vi "set led.vi"(8 "error in (no error)":errorcluster, 10 "state":i32, 11 "led":u32(ring) items=["GREEN", "RED"]) -> (0 "error out":errorcluster, 3 "function return":i32)   [LabVIEW 2014, in "libroboticscape.lvlib"]
doc: "int set_led(led_t led, int state);"
uses:
  libroboticscape.lvlib
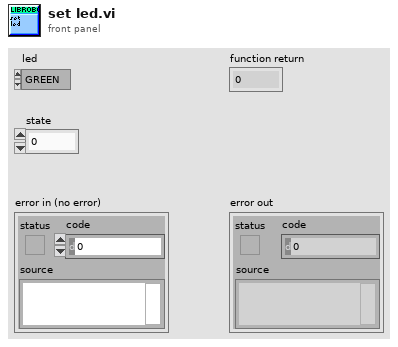
[diagram p1: front panel]
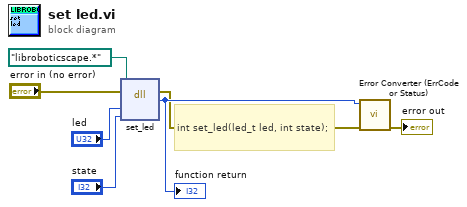
[diagram p0: block diagram]
diagram:
  # "int set_led(led_t led, int state);"
  n1 = dll-call lib="C:/Users/ktalke/Documents/Robotics-Cape-Master-Jessie/Libroboticscape-Master-Jessie/libroboticscape.so" fn="set_led"(path in=path "libroboticscape.*", error in="error in (no error)", "led"="led", "state"="state") -> (error out=w3:errorcluster, "return type"=w7:i32)  [unwired: 3 in, 1 out]
  "function return" <- w7
  n2 = call "Error Converter (ErrCode or Status).vi"("error in (no error)"=w3, "error code"=w7) -> ("error out"=→"error out":errorcluster)  [unwired: 9 in]
